vi "rad_Filter Disconnected Targets.vi"(11 "Target List Ref":refnum<vi>) -> (0 "error out":errorcluster)   [LabVIEW 2016]
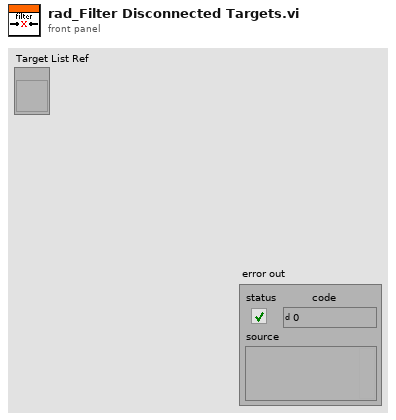
[diagram p1: front panel]
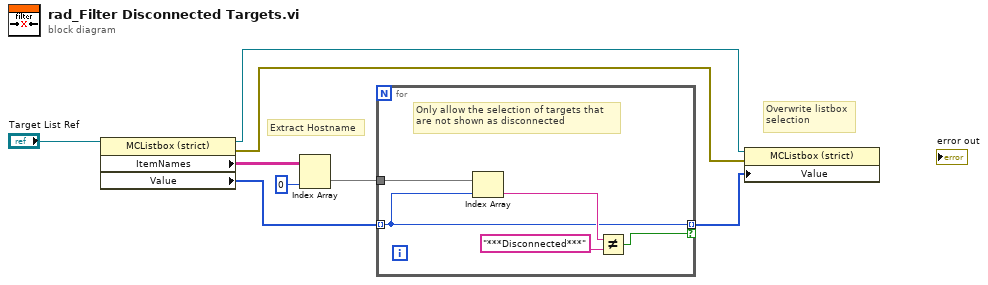
[diagram p0: block diagram]
diagram:
  # "Overwrite listbox\nselection"
  # "Extract Hostname"
  n1 = property class="MCListbox (strict)"(reference="Target List Ref") -> (reference out=w3:refnum<vi>, error out=w2:errorcluster, "ItemNames"=w6:string[][], "Value"=w7:i32[])  [unwired: 1 in]
  n2 = Index Array "Index Array"(array=w6, index (col)=0 ("disabled index (col)")) -> (element=w4:string[])  [unwired: 1 in]
  n3 = for {
    tunnel: w4 -> [w13]
    tunnel: w7 -> [w10] mode=indexing
    tunnel: [w10] -> w1 mode=indexing if=w9
    # "Only allow the selection of targets that\nare not shown as disconnected"
    n4 = Index Array "Index Array"(array=w13, index=w10) -> (element=w12:string)
    n5 = Not Equal?(x=w12, y="***Disconnected***") -> (x != y?=w9:bool)
  }
  n6 = property class="MCListbox (strict)"(reference=w3, error in=w2, "Value"=w1) -> ()  [unwired: 2 out]
